vi "Remove Capabilities.vi"(8 "error in (no error)":errorcluster, 10 "Capabilities":string[](array[string]), 11 "Node Config in":refnum<class "Node Config.lvclass">) -> (0 "error out":errorcluster, 3 "Node Config out":refnum<class "Node Config.lvclass">)   [LabVIEW 2020, in "Vecto.lvlib" / "Node Config.lvclass"]
uses:
  Node Config.lvclass
  Node Config.lvclass/Node Config.ctl
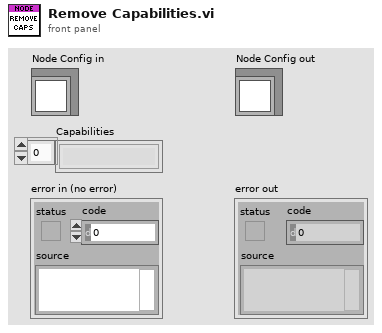
[diagram p1: front panel]
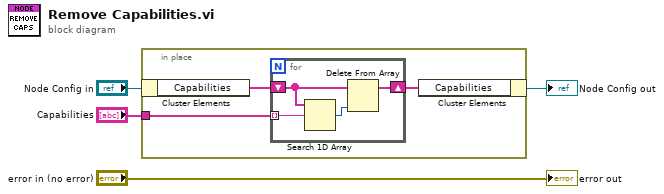
[diagram p0: block diagram]
diagram:
  n1 = in-place {
    in-place-border: "Capabilities" -> [w6]
    n2 = in-place-cluster #1("Node Config in") -> ("Capabilities"=w7:string[])
    n3 = for {
      shift-right: [w9] -> w5
      shift-left: w7 -> [w10]
      tunnel: w6 -> [w11] mode=indexing
      n4 = Search 1D Array(1D array=w10, element=w11) -> (index of element=w8:i32)  [unwired: 1 in]
      n5 = Delete From Array(array=w10, index=w8) -> (array with subset deleted=w9:string[])  [unwired: 1 in, 1 out]
    }
    n6 = in-place-cluster #1("Capabilities"=w5) -> (→"Node Config out":refnum<class "Node Config.lvclass">)
  }
  "error out" <- "error in (no error)"
